vi "scan2d_log_data.vi"(8 "error in (no error)":errorcluster, 9 "location":string, 11 "scan_2d in":refnum<class "scan_2d.lvclass">) -> (0 "error out":errorcluster, 3 "scan_2d out":refnum<class "scan_2d.lvclass">)   [LabVIEW 2015, in "scan_2d.lvclass"]
uses:
  scan_2d.lvclass
  scan_2d.lvclass/scan_2d.ctl
  scan_2d_hdf5_log/scan_2d_hdf5_log.lvclass
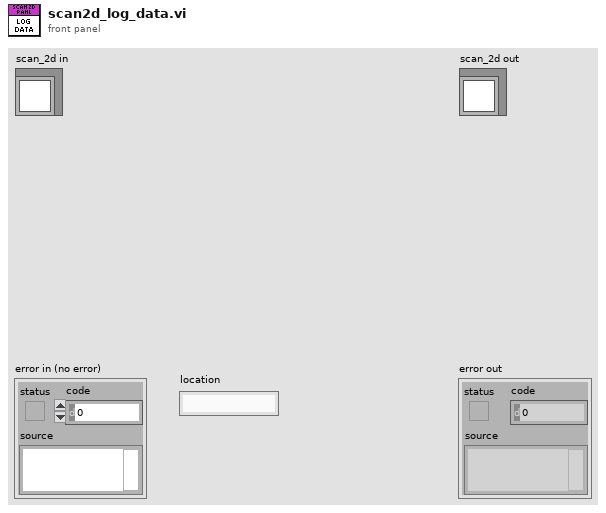
[diagram p1: front panel]
types:
  T1 = typedef "detector_data_tdef.ctl" = cluster{"data_array":dbl[][][], "data_size":cluster{"X":i32, "Y":i32, "Z":i32}}
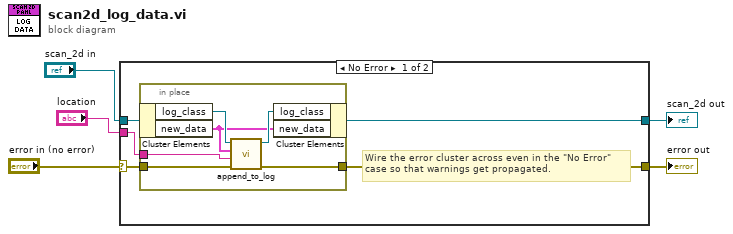
[diagram p0: block diagram]
diagram:
  n1 = case shown="No Error" "error in (no error)" {
    selector: "error in (no error)" -> [w9 w18]
    tunnel: [w8 w18] -> w4
    tunnel: [w6 w17] -> w2
    tunnel: "scan_2d in" -> [w10 w17]
    tunnel: "location" -> [w7 _]
    frame No Error {
      # "Wire the error cluster across even in the \"No Error\"\ncase so that warnings get propagated."
      n2 = in-place {
        in-place-border: w9 -> [w14]
        in-place-border: [w13] -> w8
        in-place-border: w7 -> [w12]
        n3 = in-place-cluster #1(w10) -> ("log_class"=w16:refnum<class "scan_2d_hdf5_log.lvclass">, "new_data"=w11:T1)
        n4 = call-dynamic "append_to_log.vi"("error in (no error)"=w14, "Location"=w12, "Data"=w11, "scan_hdf5_log in"=w16) -> ("error out"=w13:errorcluster, "scan_hdf5_log out"=w15:refnum<class "scan_2d_hdf5_log.lvclass">)  [unwired: 6 in]
        n5 = in-place-cluster #1("log_class"=w15, "new_data"=w11) -> (w6:refnum<class "scan_2d.lvclass">)
      }
    }
    frame Error {
    }
  }
  "error out" <- w4
  "scan_2d out" <- w2
